vi "KeysightMeasBoth.vi"(8 "error in (no error)":errorcluster, 11 "VISA resource name":refnum<visa-resource-name>="N8731APSU") -> (0 "error out":errorcluster, 1 "VOLT":dbl, 2 "CURR":dbl, 3 "VISA resource name out":refnum<visa-resource-name>)   [LabVIEW 2017]
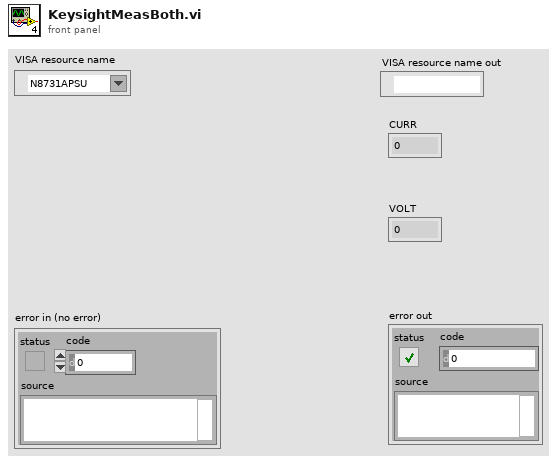
[diagram p1: front panel]
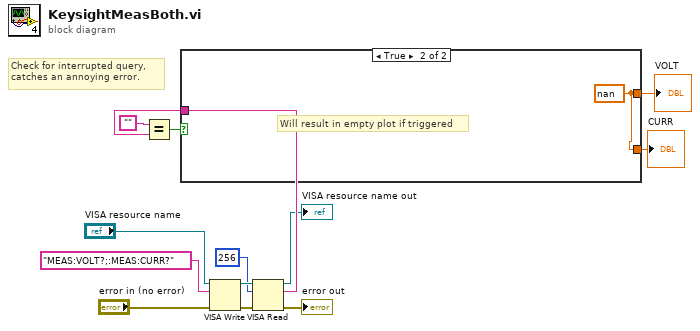
[diagram p0: block diagram]
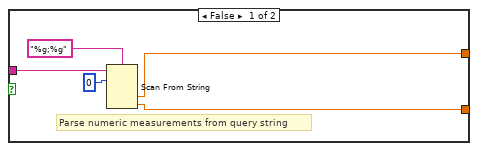
[diagram p2: hidden frame]
diagram:
  # "Check for interrupted query, \ncatches an annoying error."
  n1 = VISA Write(VISA resource name="VISA resource name", write buffer="MEAS:VOLT?;:MEAS:CURR?", error in (no error)="error in (no error)") -> (VISA resource name out=w10:refnum<visa-resource-name>, error out=w9:errorcluster)  [unwired: 1 out]
  n2 = VISA Read(VISA resource name=w10, byte count=u32 256, error in (no error)=w9) -> (VISA resource name out=→"VISA resource name out":refnum<visa-resource-name>, read buffer=w5:string, error out=→"error out":errorcluster)  [unwired: 1 out]
  n3 = Equal?(x="", y=w5) -> (x = y?=w6:bool)
  n4 = case shown="True" w6 {
    tunnel: w5 -> [w16 _]
    tunnel: [w15 w19] -> w2
    tunnel: [w14 w19] -> w1
    frame False {
      # "Parse numeric measurements from query string"
      n5 = Scan From String(format string="%g;%g", input string=w16, initial scan location=u32 0) -> (output 1=w14:dbl, output 2=w15:dbl)  [unwired: 3 in, 3 out]
    }
    frame True {
      w19 = nan
      # "Will result in empty plot if triggered"
    }
  }
  "CURR" <- w2
  "VOLT" <- w1
